vi "kleursensor implementatie.vi"() -> ()   [LabVIEW 2019]
doc: "The myRIO Project template acquires acceleration data from the onboard accelerometer and displays the changes of acceleration values in a waveform chart."
uses:
  <vilib>/myRIO/Instrument Drivers/Onboard IO/I2C/typedefs/I2C User Configuration.ctl
  <vilib>/myRIO/Instrument Drivers/Onboard IO/I2C/typedefs/I2C Transfer Rate.ctl
  <vilib>/myRIO/Instrument Drivers/Onboard IO/I2C/typedefs/I2C Reference.ctl
  <vilib>/myRIO/Common/Instrument Driver Framework/Utilities/typedefs/myRIO Generic Hardware Reference.ctl
  <vilib>/myRIO/Common/Instrument Driver Framework/Utilities/typedefs/Hardware Version Enum.ctl
  <vilib>/myRIO/Common/Instrument Driver Framework/Utilities/typedefs/myRIO v1.0 Reference.ctl
  <vilib>/myRIO/Common/Instrument Driver Framework/Utilities/typedefs/Generic FPGA Reference.ctl
  <vilib>/myRIO/Common/Instrument Driver Framework/myRIO v1.0/I2C/typedefs/I2C Channels Enum.ctl
  <vilib>/myRIO/Instrument Drivers/Onboard IO/I2C/typedefs/I2C Configuration.ctl
  <vilib>/userDefined/High Color/nirio_resource_hc.ctl
  <vilib>/myRIO/Instrument Drivers/Onboard IO/DIO/typedefs/DIO Reference.ctl
  <vilib>/myRIO/Common/Instrument Driver Framework/myRIO v1.0/DIO/typedefs/DIO Channels List.ctl
  <vilib>/myRIO/Common/Instrument Driver Framework/myRIO v1.0/DIO/typedefs/DIO Channels Enum.ctl
  <vilib>/myRIO/Common/Instrument Driver Framework/Utilities/vis/Is FPGA Ref Available.vi
  <vilib>/myRIO/Common/Instrument Driver Framework/myRIO v1.0/I2C/vis/myRIO v1.1 Open I2C.vi
  <vilib>/myRIO/Instrument Drivers/Onboard IO/I2C/vis/Configure.vi
  <vilib>/myRIO/Instrument Drivers/Onboard IO/I2C/vis/Write.vi
  <vilib>/myRIO/Common/Instrument Driver Framework/myRIO v1.0/DIO/vis/myRIO v1.1 Open DIO.vi
  <vilib>/myRIO/Instrument Drivers/Onboard IO/DIO/vis/Write.vi
  <vilib>/myRIO/Common/Instrument Driver Framework/Utilities/vis/Validate Channels.vi
  <vilib>/myRIO/Common/Instrument Driver Framework/myRIO v1.0/I2C/vis/myRIO v1.0 Reserve I2C.vi
  <vilib>/myRIO/Common/Instrument Driver Framework/myRIO v1.0/DIO/vis/myRIO v1.0 Reserve DIO.vi
  <vilib>/myRIO/Common/Instrument Driver Framework/myRIO v1.0/I2C/vis/myRIO v1.0 Build MUX Configuration I2C.vi
  <vilib>/myRIO/Common/Instrument Driver Framework/myRIO v1.0/Resource Manager/vis/myRIO v1.0 Reserve Channel List.vi
  <vilib>/myRIO/Common/Instrument Driver Framework/myRIO v1.0/DIO/vis/myRIO v1.0 Build MUX Configuration DIO.vi
  <vilib>/myRIO/Common/Instrument Driver Framework/myRIO v1.0/Resource Manager/vis/myRIO v1.0 Create Configuration List.vi
  <vilib>/myRIO/Common/Instrument Driver Framework/myRIO v1.0/Resource Manager/vis/myRIO v1.0 Reserve Channel.vi
  <vilib>/myRIO/Common/Instrument Driver Framework/myRIO v1.0/Resource Manager/vis/myRIO v1.0 Unreserve Channel.vi
  <vilib>/myRIO/Common/Instrument Driver Framework/myRIO v1.0/Resource Manager/vis/myRIO v1.0 Build Mutex Name.vi
  <vilib>/Utility/VariantDataType/GetNumericInfo.vi
  <vilib>/Utility/error.llb/Error Cluster From Error Code.vi
  <vilib>/myRIO/Common/Instrument Driver Framework/myRIO v1.0/myRIO v1.1 Open.vi
  <vilib>/myRIO/Common/Instrument Driver Framework/Utilities/vis/IO Manager.vi
  <vilib>/myRIO/Common/Instrument Driver Framework/Utilities/vis/Configuration Manager.vi
  <vilib>/myRIO/Common/Instrument Driver Framework/myRIO v1.0/Resource Manager/vis/myRIO v1.0 Configure IO.vi
  <vilib>/myRIO/Common/Instrument Driver Framework/myRIO v1.0/myRIO v1.0 Close.vi
  <vilib>/myRIO/Common/Instrument Driver Framework/myRIO v1.0/DIO/vis/myRIO v1.0 Write DIO.vi
  <vilib>/myRIO/Common/Instrument Driver Framework/myRIO v1.0/I2C/vis/myRIO v1.0 Configure I2C.vi
  <vilib>/myRIO/Common/Instrument Driver Framework/myRIO v1.0/I2C/vis/myRIO v1.0 Write I2C.vi
  <vilib>/myRIO/Express VI/Onboard IO/DO/DO Express VI.xnode
  <vilib>/myRIO/Instrument Drivers/Onboard IO/DIO/vis/myRIO DIO Open.xnode
  <vilib>/myRIO/Express VI/Onboard IO/I2C/I2C Express VI.xnode
  <vilib>/myRIO/Instrument Drivers/Onboard IO/I2C/vis/myRIO I2C Open.xnode
  <vilib>/myRIO/Instrument Drivers/Onboard IO/DIO/DIO.lvlib
  <vilib>/myRIO/Instrument Drivers/Onboard IO/I2C/I2C.lvlib
panel:
  out "rood 2":i32[](array[numeric])
  out "groen":i32[](array[numeric])
  out "error out 3":errorcluster
  in  "error in (no error) 3":errorcluster
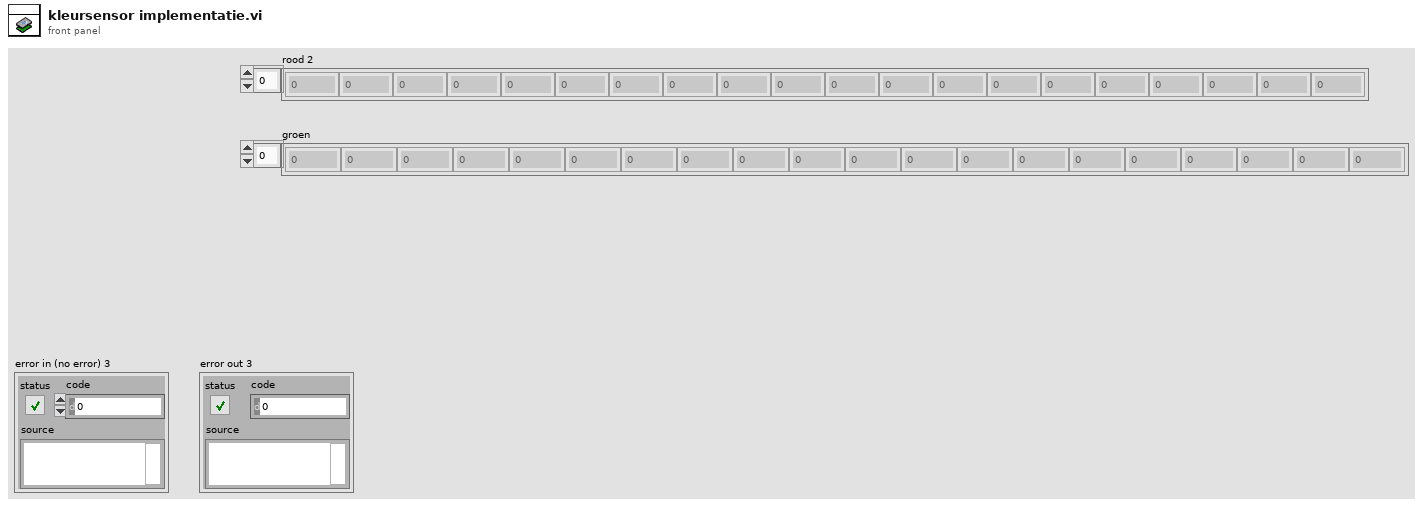
[diagram p1: front panel]
types:
  T1 = typedef "I2C.lvlib/I2C Reference.ctl" = cluster{"myRIO Reference":T2, "I2C Channels Enum":T6, "I2C Configuration":T7}
  T2 = typedef "myRIO Generic Hardware Reference.ctl" = cluster{"myRIO Model":T3, "myRIO Hardware Reference":T4}
  T3 = typedef "Hardware Version Enum.ctl" = enum16{"Unknown", "myRIO-1900", "myRIO-1950", "roboRIO", "NI ELVIS RIO CM", "ELVIS III"}
  T4 = typedef "myRIO v1.0 Reference.ctl" = cluster{"Generic FPGA Reference":T5, "Allow multiple opens":bool}
  T5 = typedef "Generic FPGA Reference.ctl" = refnum<k20>
  T6 = typedef "I2C Channels Enum.ctl" = enum16{"Not Connected", "A/I2C", "B/I2C", "I2C/I2C"}
  T7 = typedef "I2C.lvlib/I2C Configuration.ctl" = cluster{"I2C Transfer Rate":T8}
  T8 = typedef "I2C.lvlib/I2C Transfer Rate.ctl" = enum16{"Standard mode (100 kbps)", "Fast mode (400 kbps)"}
  T9 = typedef "I2C.lvlib/I2C User Configuration.ctl" = cluster{"I2C Transfer Rate":T8}
  T10 = typedef "nirio_resource_hc.ctl" = tag
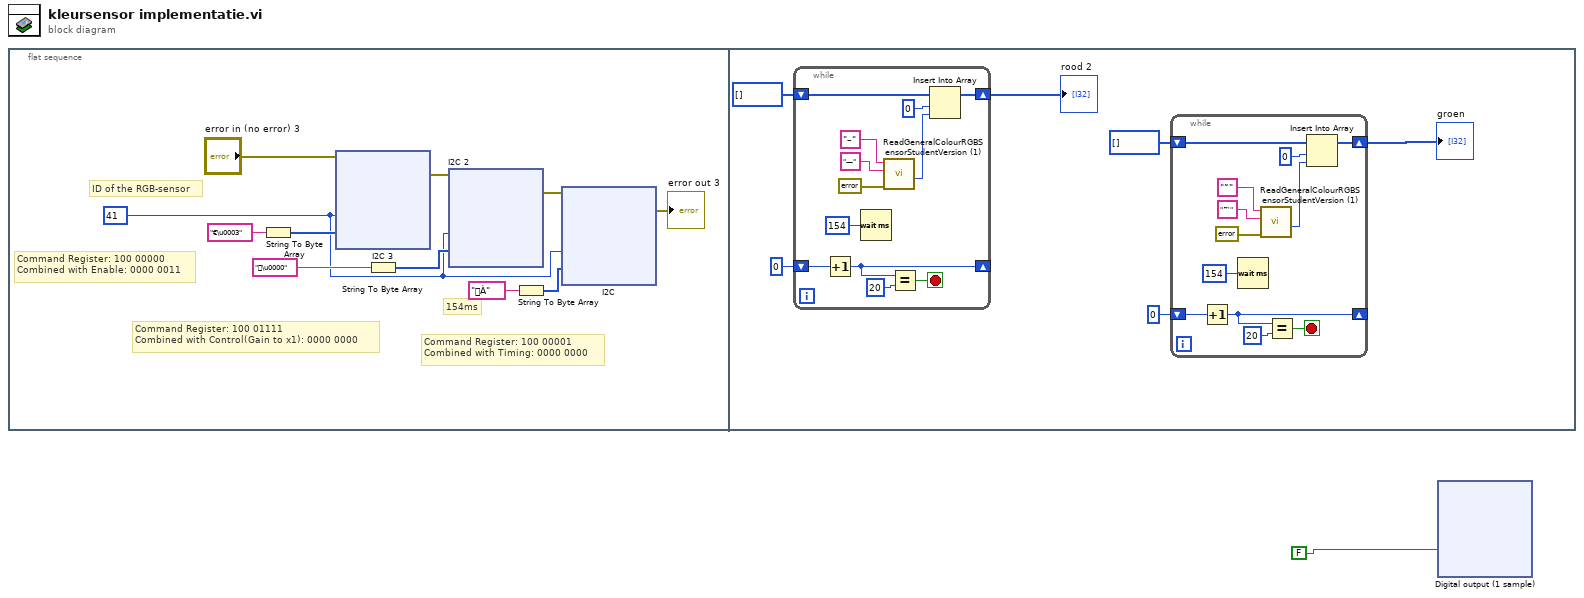
[diagram p0: block diagram]
diagram:
  n1 = flat-sequence {
    frame #0 {
      w6 = 41 ("Numeric")
      # "154ms"
      # "ID of the RGB-sensor"
      # "Command Register: 100 00000\nCombined with Enable: 0000 0011"
      # "Command Register: 100 01111\nCombined with Control(Gain to x1): 0000 0000"
      # "Command Register: 100 00001\nCombined with Timing: 0000 0000"
      n2 = String To Byte Array(string="€\u0003") -> (unsigned byte array=w9:u8[])
      n3 = xnode "I2C 3"("Slave Address (7-bit)"=w6, "Bytes to Write"=w9, "error in (no error)"="error in (no error) 3") -> ("error out"=w5:errorcluster)
      n4 = String To Byte Array(string="\u0000") -> (unsigned byte array=w8:u8[])
      n5 = xnode "I2C 2"("Slave Address (7-bit)"=w6, "Bytes to Write"=w8, "error in (no error)"=w5) -> ("error out"=w4:errorcluster)
      n6 = String To Byte Array(string="À") -> (unsigned byte array=w7:u8[])
      n7 = xnode "I2C"("Slave Address (7-bit)"=w6, "Bytes to Write"=w7, "error in (no error)"=w4) -> ("error out"=→"error out 3":errorcluster)
    }
    frame #1 {
      n8 = while {
        shift-right: [w150] -> w130
        shift-left: i32[] [] -> [w149]
        shift-right: [w146] -> _
        shift-left: 0 -> [w148]
        stop <- w147 stop-if-true
        n9 = Increment(x=w148) -> (x+1=w146:i32)
        n10 = Wait (ms)(milliseconds to wait=u32 154) -> ()  [unwired: 1 out]
        n11 = call "ReadGeneralColourRGBSensorStudentVersion (1).vi"("error in (no error)"=errorcluster {"status"=FALSE, "code"=0, "source"=""}, "High"="—", "Low"="–") -> ("Total"=w152:u32)  [unwired: 5 in, 3 out]
        n12 = Equal?(x=w146, y=20) -> (x = y?=w147:bool)
        n13 = Insert Into Array(array=w149, index=0, new element=w152) -> (w150:i32[])
      }
      "rood 2" <- w130
      n14 = while {
        shift-right: [w138] -> w127
        shift-left: i32[] [] -> [w137]
        shift-right: [w134] -> _
        shift-left: 0 -> [w136]
        stop <- w135 stop-if-true
        n15 = Increment(x=w136) -> (x+1=w134:i32)
        n16 = Wait (ms)(milliseconds to wait=u32 154) -> ()  [unwired: 1 out]
        n17 = call "ReadGeneralColourRGBSensorStudentVersion (1).vi"("error in (no error)"=errorcluster {"status"=FALSE, "code"=0, "source"=""}, "High"="™", "Low"="˜") -> ("Total"=w140:u32)  [unwired: 5 in, 3 out]
        n18 = Equal?(x=w134, y=20) -> (x = y?=w135:bool)
        n19 = Insert Into Array(array=w137, index=0, new element=w140) -> (w138:i32[])
      }
      "groen" <- w127
    }
  }
  n20 = xnode "Digital output (1 sample)"("A/DIO2 (Pin 15)"=FALSE) -> ()  [unwired: 1 in, 1 out]
